vi "HistogramManual2004.vi"   [LabVIEW 2013]
uses:
  <vilib>/Heliosphere Research LLC/Advanced Plotting Toolkit/api_plotting/HistogramProperties.ctl
  <vilib>/Heliosphere Research LLC/Advanced Plotting Toolkit/typedefs/PlotColor.ctl
  <vilib>/Heliosphere Research LLC/Advanced Plotting Toolkit/properties/Line.ctl
  <vilib>/Heliosphere Research LLC/Advanced Plotting Toolkit/properties/Line_Style.ctl
  <vilib>/Heliosphere Research LLC/Advanced Plotting Toolkit/properties/Display.ctl
  <vilib>/Heliosphere Research LLC/Advanced Plotting Toolkit/api_plotting/Histogram_Manual.vi
  <vilib>/Heliosphere Research LLC/Advanced Plotting Toolkit/Advanced Plotting Toolkit.lvlib
types:
  T1 = typedef "Advanced Plotting Toolkit.lvlib/HistogramProperties.ctl" = cluster{"Color":T2, "Cumulative":bool, "Normalize":bool, "Line":T3, "Display":T5}
  T2 = typedef "Advanced Plotting Toolkit.lvlib/PlotColor.ctl" = u32
  T3 = typedef "Advanced Plotting Toolkit.lvlib/Line.ctl" = cluster{"Style":T4, "Color":T2, "Width":sgl}
  T4 = typedef "Advanced Plotting Toolkit.lvlib/Line_Style.ctl" = enum16{"Automatic", "Solid", "Dashed", "Dotted", "Dash-dot", "Invisible"}
  T5 = typedef "Advanced Plotting Toolkit.lvlib/Display.ctl" = cluster{"Alpha":dbl, "Z Order":dbl}
  T6 = typedef "Advanced Plotting Toolkit.lvlib/PlotID.ctl" = i32
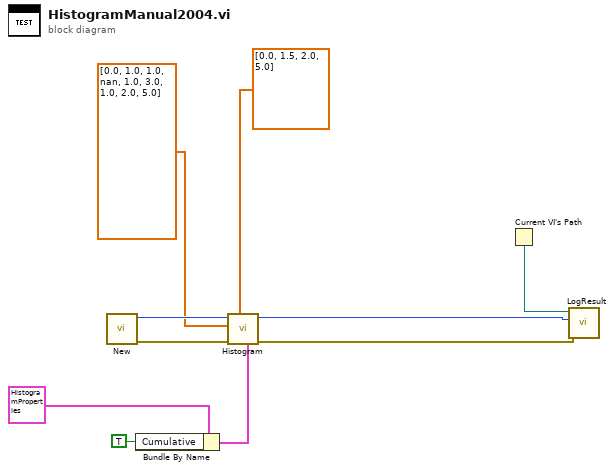
[diagram p0: block diagram]
diagram:
  n1 = call <vilib>:"New.vi"() -> ("error out"=w7:errorcluster, "Plot ID"=w10:T6)  [unwired: 10 in]
  n2 = Bundle By Name(cluster=T1 {"Color"=2147483647, "Cumulative"=FALSE, "Normalize"=FALSE, "Line"={"Style"=enum."Automatic", "Color"=2147483647, "Width"=nan}, "Display"={"Alpha"=nan, "Z Order"=nan}} ("Histogram Properties"), "Cumulative"=TRUE) -> (w3:T1)
  n3 = call-poly <vilib>:"Histogram.vi"("Properties"=w3, "Bins"=dbl[] [0.0, 1.5, 2.0, 5.0], "error in (no error)"=w7, "Data"=dbl[] [0.0, 1.0, 1.0, nan, 1.0, 3.0, 1.0, 2.0, 5.0], "Plot ID"=w10) -> ("error out"=w6:errorcluster, "Plot ID Out"=w9:T6)  [unwired: 5 in]
  n4 = Current VI's Path() -> (path=w8:path)
  n5 = call "LogResult.vi"("Test Result"=w6, "Test Artifact"=w9, "VI Path"=w8) -> ()  [unwired: 9 in]
